vi "sub_save output files.vi"(3 "Raw Queue in":refnum<queue>, 4 "Processed Queue in":refnum<queue>, 6 "Raw Data error":errorcluster, 7 "Processed Data error":errorcluster) -> (5 "error out":errorcluster)   [LabVIEW 2020]
uses:
  globalvariables.vi
  <vilib>/Utility/file.llb/Write Delimited Spreadsheet (DBL).vi
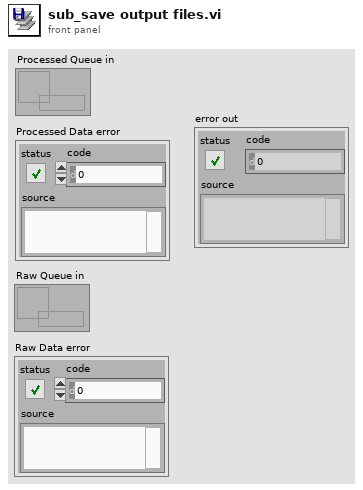
[diagram p1: front panel]
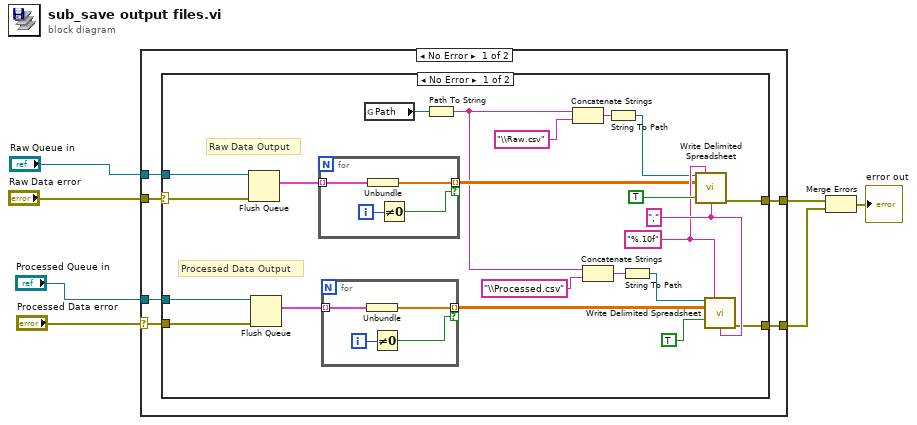
[diagram p0: block diagram]
diagram:
  n1 = case shown="No Error" "Processed Data error" {
    selector: "Processed Data error" -> [w12 w46]
    tunnel: "Processed Queue in" -> [w13 _]
    tunnel: "Raw Queue in" -> [w11 _]
    tunnel: "Raw Data error" -> [w10 w47]
    tunnel: [w9 w47] -> w3
    tunnel: [w8 w46] -> w2
    frame No Error {
      n2 = case shown="No Error" w10 {
        selector: w10 -> [w21 w45]
        tunnel: w13 -> [w31 _]
        tunnel: w12 -> [w30 w44]
        tunnel: w11 -> [w22 _]
        tunnel: [w17 w45] -> w9
        tunnel: [w16 w44] -> w8
        frame No Error {
          w32 = "%.10f"
          w33 = ","
          # "Raw Data Output"
          # "Processed Data Output"
          n3 = Flush Queue(queue=w22, error in (no error)=w21) -> (remaining elements=w23:cluster{dbl[]}[])  [unwired: 2 out]
          n4 = Flush Queue(queue=w31, error in (no error)=w30) -> (remaining elements=w15:cluster{dbl[]}[])  [unwired: 2 out]
          n5 = for {
            tunnel: w23 -> [w43] mode=indexing
            tunnel: [w42] -> w20 mode=indexing if=w40
            i -> [w41]
            n6 = Unbundle(w43) -> (w42:dbl[])
            n7 = Not Equal To 0?(x=w41) -> (x != 0?=w40:bool)
          }
          n8 = for {
            tunnel: w15 -> [w39] mode=indexing
            tunnel: [w38] -> w14 mode=indexing if=w36
            i -> [w37]
            n9 = Unbundle(w39) -> (w38:dbl[])
            n10 = Not Equal To 0?(x=w37) -> (x != 0?=w36:bool)
          }
          n11 = global read "globalvariables.vi" "Path"() -> (w24:path)
          n12 = Path To String(path=w24) -> (string=w19:string)
          n13 = Concatenate Strings(w19, "\\Raw.csv") -> (w28:string)
          n14 = Concatenate Strings(w19, "\\Processed.csv") -> (w29:string)
          n15 = String To Path(string=w28) -> (path=w18:path)
          n16 = String To Path(string=w29) -> (path=w25:path)
          n17 = call-poly <vilib>:"Write Delimited Spreadsheet.vi"("file path (dialog if empty)"=w18, "format (%.3f)"=w32, "2D data"=w20, "append to file? (new file:F)"=TRUE, "delimiter (\\t)"=w33) -> ("error out"=w17:errorcluster)  [unwired: 9 in, 1 out]
          n18 = call-poly <vilib>:"Write Delimited Spreadsheet.vi"("file path (dialog if empty)"=w25, "format (%.3f)"=w32, "2D data"=w14, "append to file? (new file:F)"=TRUE, "delimiter (\\t)"=w33) -> ("error out"=w16:errorcluster)  [unwired: 9 in, 1 out]
        }
        frame Error {
        }
      }
    }
    frame Error {
    }
  }
  n19 = Merge Errors(w3, w2) -> (→"error out":errorcluster)
